vi "Finish.vi"   [LabVIEW 2017]
doc: "This VI is called just before exiting. It is expected to close I/O refnum, save collected data, etc."
uses:
  <vilib>/Rock Robotics/WPI/Utilities/WPI_GetSetVariantRefNum.vi
types:
  T1 = typedef "WPI_JoystickDevRef.ctl" = cluster{"Device":T2}
  T2 = typedef "WPI_JoystickDeviceEnum.ctl" = enum16{"USB 0", "USB 1", "USB 2", "USB 3", "USB 4", "USB 5"}
  T3 = typedef "WPI_DigitalInputDevRef.ctl" = cluster{"DevStatus":errorcluster, "DIO Channel":T4}
  T4 = typedef "FPGA_DIOChannel.ctl" = enum8{"DIO 0", "DIO 1", "DIO 2", "DIO 3", "DIO 4", "DIO 5", "DIO 6", "DIO 7", "DIO 8", "DIO 9", "DIO MXP 0", "DIO MXP 1", "DIO MXP 2", "DIO MXP 3", "DIO MXP 4", "DIO MXP 5", "DIO MXP 6", "DIO MXP 7", "DIO MXP 8", "DIO MXP 9", "DIO MXP 10", "DIO MXP 11", "DIO MXP 12", "DIO MXP 13", "DIO MXP 14", "DIO MXP 15", "SPI Port CS1", "SPI Port CS2", "SPI Port CS3", "SPI Port MISO", "SPI Port MOSI", "Invalid"}
  T5 = typedef "WPI_RobotDriveDevRef.ctl" = cluster{"DevStatus":errorcluster, "Motors[]":T6[], "Square Inputs":bool, "Max Output":dbl}
  T6 = typedef "WPI_MotorControlDeviceRef.ctl" = cluster{"DeviceStatus":errorcluster, "Type":T7, "PWM":cluster{"PWM Channel":T8, "DeadBand":T9}, "CAN":cluster{"Device Number":u8, "SetOutput VI Ref":variant, "GetOutput VI Ref":variant, "Enable VI Ref":variant, "Disable VI Ref":variant, "Data":variant}, "Invert":bool, "DIO PWM":cluster{"PWM \"Enable\" Channel":T8, "DIOChannel":T4, "PWM Rate":dbl}}
  T7 = typedef "WPI_MotorControlType.ctl" = enum16{"PWM", "CAN", "DIO PWM"}
  T8 = typedef "FPGA_DIOPWMChannel.ctl" = enum8{"PWM 0", "PWM 1", "PWM 2", "PWM 3", "PWM 4", "PWM 5", "PWM 6", "PWM 7", "PWM 8", "PWM 9", "PWM MXP 0", "PWM MXP 1", "PWM MXP 2", "PWM MXP 3", "PWM MXP 4", "PWM MXP 5", "PWM MXP 6", "PWM MXP 7", "PWM MXP 8", "PWM MXP 9", "Invalid"}
  T9 = typedef "WPI_PWMDeadband.ctl" = cluster{"Name":string, "maxPositivePwm":i32, "minPositivePwm":i32, "centerPwm":i32, "maxNegativePwm":i32, "minNegativePwm":i32, "angularRange":u16}
  T10 = typedef "WPI_SolenoidDevRef.ctl" = cluster{"DevStatus":errorcluster, "Pneumatics Control Module":u8, "Forward Solenoid Channel":T11, "Reverse Solenoid Channel":T11}
  T11 = typedef "WPI_SolenoidChannel.ctl" = enum8{"Solenoid 0", "Solenoid 1", "Solenoid 2", "Solenoid 3", "Solenoid 4", "Solenoid 5", "Solenoid 6", "Solenoid 7", "Invalid"}
  T12 = typedef "WPI_EncoderDevRef.ctl" = cluster{"DevStatus":errorcluster, "EncoderIndex":T13, "CounterIndex":T14, "DistancePerCount":dbl, "Decoding Type":T15}
  T13 = typedef "FPGA_EncoderIdx.ctl" = enum8{"Enc 0", "Enc 1", "Enc 2", "Enc 3", "Enc 4", "Enc 5", "Enc 6", "Enc 7", "Invalid"}
  T14 = typedef "FPGA_CounterCtrSystemIndex.ctl" = enum8{"Ctr 0", "Ctr 1", "Ctr 2", "Ctr 3", "Ctr 4", "Ctr 5", "Ctr 6", "Ctr 7", "Invalid"}
  T15 = typedef "WPI_EncoderType.ctl" = enum16{"1x", "2x", "4x"}
  T16 = typedef "WPI_CompressorDevRef.ctl" = cluster{"DevStatus":errorcluster, "Pneumatics Control Module":u8}
  T17 = typedef "WPI_SwitchDevRef.ctl" = cluster{"DevStatus":errorcluster, "DIO Channel":T4, "CntIndex":T14, "Normally Closed":bool}
  T18 = typedef "WPI_GyroDevRef.ctl" = cluster{"DevStatus":errorcluster, "Analog Channel":T19, "Gain (VoltsPerDegree/Second)":dbl, "Gyro Type":enum16{"Analog", "XRS450"}, "Handle":i32, "SPI Bus":T20, "Device Found":bool, "Sample Rate":dbl, "Calibrate On Open":bool, "Offset":dbl}
  T19 = typedef "FPGA_AIChannel.ctl" = enum8{"AI 0", "AI 1", "AI 2", "AI 3", "AI MXP 0", "AI MXP 1", "AI MXP 2", "AI MXP 3", "Invalid"}
  T20 = typedef "spi_bus.ctl" = enum16{"SPI On-Board, CS0", "SPI On-Board, CS1", "SPI On-Board, CS2", "SPI On-Board, CS3", "SPI MXP", "Invalid"}
  T21 = typedef "WPI_RelayDevRef.ctl" = cluster{"DevStatus":errorcluster, "Relay Channel":T22, "Relay Direction":T23}
  T22 = typedef "FPGA_DIORelayChannel.ctl" = enum8{"Relay 0", "Relay 1", "Relay 2", "Relay 3", "Invalid"}
  T23 = typedef "WPI_RelayDirection.ctl" = enum16{"Both directions", "Forward only", "Reverse only"}
  T24 = typedef "WPI_AnalogChannelDevRef.ctl" = cluster{"DevStatus":errorcluster, "Analog Channel":T19}
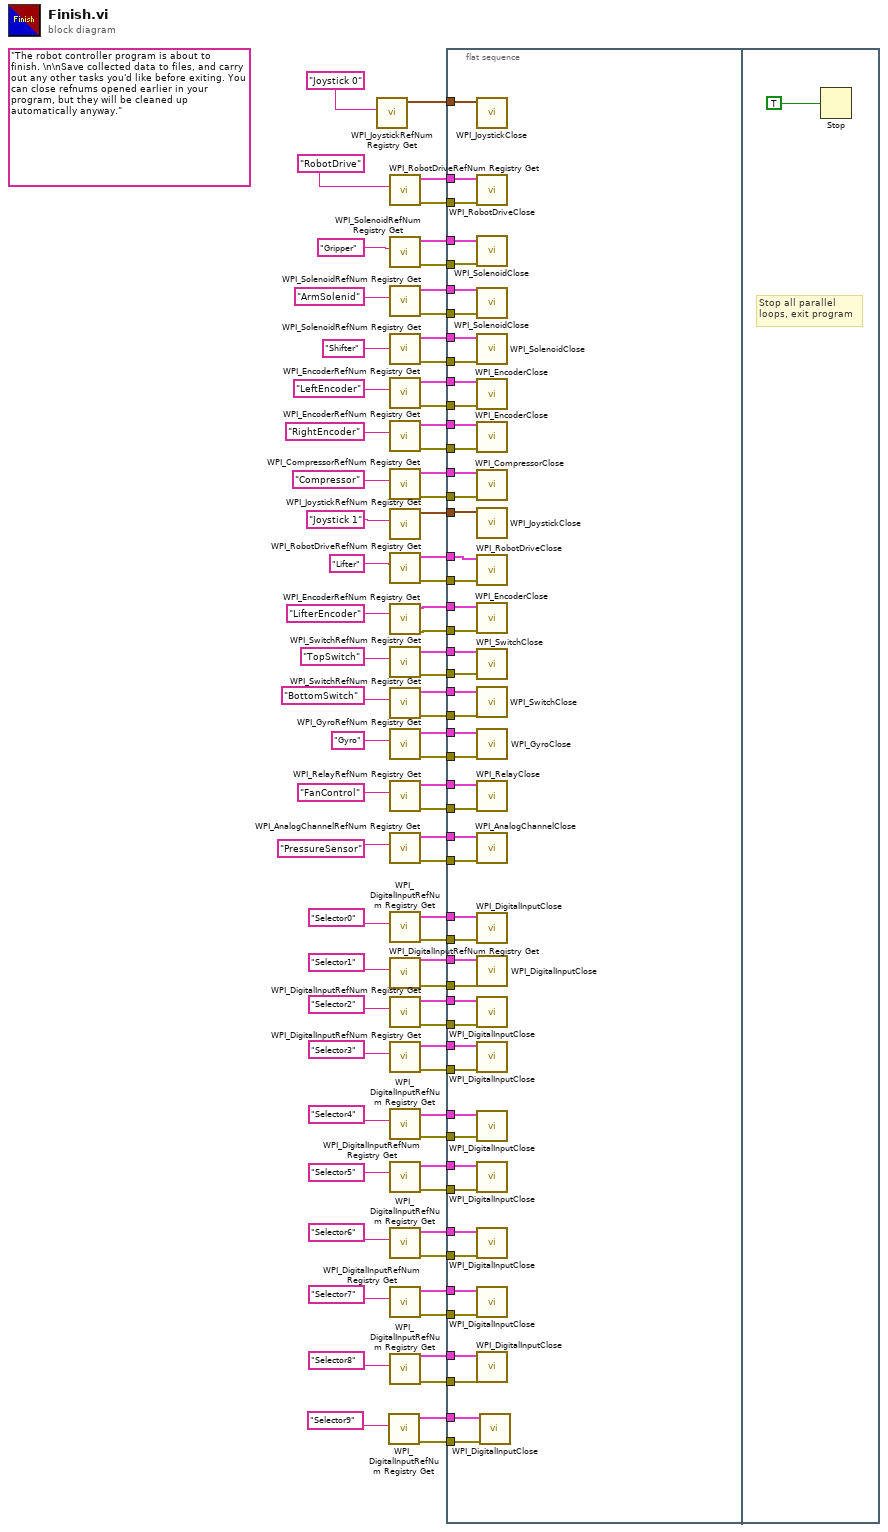
[diagram p0: block diagram]
diagram:
  (unwired) "The robot controller program is about to finish. \n\nSave collected data to files, and carry out any other tasks you'd like before exiting. You can close refnums opened earlier in your program, but they will be cleaned up automatically anyway."
  n1 = call <vilib>:"WPI_JoystickRefNum Registry Get.vi"("refnum name"="Joystick 0") -> ("JoystickDevRef"=w73:T1)  [unwired: 1 in, 9 out]
  n2 = call <vilib>:"WPI_DigitalInputRefNum Registry Get.vi"("refnum name"="Selector9") -> ("error out"=w1:errorcluster, "DigitalInputDevRef"=w2:T3)  [unwired: 9 in]
  n3 = call <vilib>:"WPI_RobotDriveRefNum Registry Get.vi"("refnum name"="RobotDrive") -> ("error out"=w34:errorcluster, "RobotDriveDevRef"=w74:T5)  [unwired: 1 in, 8 out]
  n4 = call <vilib>:"WPI_SolenoidRefNum Registry Get.vi"("refnum name"="Gripper") -> ("error out"=w65:errorcluster, "SolenoidDevRef"=w64:T10)  [unwired: 9 in]
  n5 = call <vilib>:"WPI_SolenoidRefNum Registry Get.vi"("refnum name"="ArmSolenid") -> ("error out"=w67:errorcluster, "SolenoidDevRef"=w66:T10)  [unwired: 9 in]
  n6 = call <vilib>:"WPI_SolenoidRefNum Registry Get.vi"("refnum name"="Shifter") -> ("error out"=w69:errorcluster, "SolenoidDevRef"=w68:T10)  [unwired: 9 in]
  n7 = call <vilib>:"WPI_EncoderRefNum Registry Get.vi"("refnum name"="LeftEncoder") -> ("error out"=w63:errorcluster, "EncoderDevRef"=w62:T12)  [unwired: 9 in]
  n8 = call <vilib>:"WPI_EncoderRefNum Registry Get.vi"("refnum name"="RightEncoder") -> ("error out"=w61:errorcluster, "EncoderDevRef"=w60:T12)  [unwired: 9 in]
  n9 = call <vilib>:"WPI_CompressorRefNum Registry Get.vi"("refnum name"="Compressor") -> ("error out"=w57:errorcluster, "CompressorDevRef"=w56:T16)  [unwired: 9 in]
  n10 = call <vilib>:"WPI_JoystickRefNum Registry Get.vi"("refnum name"="Joystick 1") -> ("JoystickDevRef"=w53:T1)  [unwired: 9 in, 1 out]
  n11 = call <vilib>:"WPI_RobotDriveRefNum Registry Get.vi"("refnum name"="Lifter") -> ("error out"=w35:errorcluster, "RobotDriveDevRef"=w52:T5)  [unwired: 9 in]
  n12 = call <vilib>:"WPI_EncoderRefNum Registry Get.vi"("refnum name"="LifterEncoder") -> ("error out"=w48:errorcluster, "EncoderDevRef"=w49:T12)  [unwired: 9 in]
  n13 = call <vilib>:"WPI_SwitchRefNum Registry Get.vi"("refnum name"="TopSwitch") -> ("error out"=w46:errorcluster, "SwitchDevRef"=w47:T17)  [unwired: 9 in]
  n14 = call <vilib>:"WPI_SwitchRefNum Registry Get.vi"("refnum name"="BottomSwitch") -> ("error out"=w43:errorcluster, "SwitchDevRef"=w44:T17)  [unwired: 9 in]
  n15 = call <vilib>:"WPI_GyroRefNum Registry Get.vi"("refnum name"="Gyro") -> ("error out"=w41:errorcluster, "GyroDevRef"=w40:T18)  [unwired: 9 in]
  n16 = call <vilib>:"WPI_RelayRefNum Registry Get.vi"("refnum name"="FanControl") -> ("error out"=w37:errorcluster, "RelayDevRef"=w38:T21)  [unwired: 9 in]
  n17 = call <vilib>:"WPI_AnalogChannelRefNum Registry Get.vi"("refnum name"="PressureSensor") -> ("error out"=w31:errorcluster, "AIDeviceRef"=w32:T24)  [unwired: 9 in]
  n18 = call <vilib>:"WPI_DigitalInputRefNum Registry Get.vi"("refnum name"="Selector0") -> ("error out"=w29:errorcluster, "DigitalInputDevRef"=w30:T3)  [unwired: 9 in]
  n19 = call <vilib>:"WPI_DigitalInputRefNum Registry Get.vi"("refnum name"="Selector1") -> ("error out"=w18:errorcluster, "DigitalInputDevRef"=w19:T3)  [unwired: 9 in]
  n20 = call <vilib>:"WPI_DigitalInputRefNum Registry Get.vi"("refnum name"="Selector2") -> ("error out"=w16:errorcluster, "DigitalInputDevRef"=w17:T3)  [unwired: 9 in]
  n21 = call <vilib>:"WPI_DigitalInputRefNum Registry Get.vi"("refnum name"="Selector3") -> ("error out"=w14:errorcluster, "DigitalInputDevRef"=w15:T3)  [unwired: 9 in]
  n22 = call <vilib>:"WPI_DigitalInputRefNum Registry Get.vi"("refnum name"="Selector4") -> ("error out"=w12:errorcluster, "DigitalInputDevRef"=w13:T3)  [unwired: 9 in]
  n23 = call <vilib>:"WPI_DigitalInputRefNum Registry Get.vi"("refnum name"="Selector5") -> ("error out"=w10:errorcluster, "DigitalInputDevRef"=w11:T3)  [unwired: 9 in]
  n24 = call <vilib>:"WPI_DigitalInputRefNum Registry Get.vi"("refnum name"="Selector6") -> ("error out"=w8:errorcluster, "DigitalInputDevRef"=w9:T3)  [unwired: 9 in]
  n25 = call <vilib>:"WPI_DigitalInputRefNum Registry Get.vi"("refnum name"="Selector7") -> ("error out"=w6:errorcluster, "DigitalInputDevRef"=w7:T3)  [unwired: 9 in]
  n26 = call <vilib>:"WPI_DigitalInputRefNum Registry Get.vi"("refnum name"="Selector8") -> ("error out"=w4:errorcluster, "DigitalInputDevRef"=w5:T3)  [unwired: 9 in]
  n27 = flat-sequence {
    tunnel: w74 -> [w126]
    tunnel: w73 -> [w125]
    tunnel: w69 -> [w124]
    tunnel: w68 -> [w123]
    tunnel: w67 -> [w122]
    tunnel: w66 -> [w121]
    tunnel: w65 -> [w120]
    tunnel: w64 -> [w119]
    tunnel: w63 -> [w118]
    tunnel: w62 -> [w117]
    tunnel: w61 -> [w116]
    tunnel: w60 -> [w115]
    tunnel: w57 -> [w114]
    tunnel: w56 -> [w113]
    tunnel: w53 -> [w112]
    tunnel: w52 -> [w111]
    tunnel: w49 -> [w110]
    tunnel: w48 -> [w109]
    tunnel: w47 -> [w108]
    tunnel: w46 -> [w107]
    tunnel: w44 -> [w106]
    tunnel: w43 -> [w105]
    tunnel: w41 -> [w104]
    tunnel: w40 -> [w103]
    tunnel: w38 -> [w102]
    tunnel: w37 -> [w101]
    tunnel: w35 -> [w100]
    tunnel: w34 -> [w99]
    tunnel: w32 -> [w98]
    tunnel: w31 -> [w97]
    tunnel: w30 -> [w96]
    tunnel: w29 -> [w95]
    tunnel: w19 -> [w94]
    tunnel: w18 -> [w93]
    tunnel: w17 -> [w92]
    tunnel: w16 -> [w91]
    tunnel: w15 -> [w90]
    tunnel: w14 -> [w89]
    tunnel: w13 -> [w88]
    tunnel: w12 -> [w87]
    tunnel: w11 -> [w86]
    tunnel: w10 -> [w85]
    tunnel: w9 -> [w84]
    tunnel: w8 -> [w83]
    tunnel: w7 -> [w82]
    tunnel: w6 -> [w81]
    tunnel: w5 -> [w80]
    tunnel: w4 -> [w79]
    tunnel: w2 -> [w78]
    tunnel: w1 -> [w77]
    frame #0 {
      n28 = call <vilib>:"WPI_JoystickClose.vi"("JoystickDevRef"=w125) -> ()  [unwired: 11 out]
      n29 = call <vilib>:"WPI_RobotDriveClose.vi"("error in (no error)"=w99, "RobotDriveDevRef"=w126) -> ()  [unwired: 10 out]
      n30 = call <vilib>:"WPI_SolenoidClose.vi"("error in (no error)"=w120, "SolenoidDevRef"=w119) -> ()  [unwired: 9 in, 1 out]
      n31 = call <vilib>:"WPI_SolenoidClose.vi"("error in (no error)"=w122, "SolenoidDevRef"=w121) -> ()  [unwired: 9 in, 1 out]
      n32 = call <vilib>:"WPI_SolenoidClose.vi"("error in (no error)"=w124, "SolenoidDevRef"=w123) -> ()  [unwired: 9 in, 1 out]
      n33 = call <vilib>:"WPI_EncoderClose.vi"("error in (no error)"=w118, "EncoderDevRef"=w117) -> ()  [unwired: 9 in, 1 out]
      n34 = call <vilib>:"WPI_EncoderClose.vi"("error in (no error)"=w116, "EncoderDevRef"=w115) -> ()  [unwired: 9 in, 1 out]
      n35 = call <vilib>:"WPI_CompressorClose.vi"("error in (no error)"=w114, "CompressorDevRef"=w113) -> ()  [unwired: 9 in, 1 out]
      n36 = call <vilib>:"WPI_JoystickClose.vi"("JoystickDevRef"=w112) -> ()  [unwired: 11 out]
      n37 = call <vilib>:"WPI_RobotDriveClose.vi"("error in (no error)"=w100, "RobotDriveDevRef"=w111) -> ()  [unwired: 9 in, 1 out]
      n38 = call <vilib>:"WPI_EncoderClose.vi"("error in (no error)"=w109, "EncoderDevRef"=w110) -> ()  [unwired: 9 in, 1 out]
      n39 = call <vilib>:"WPI_SwitchClose.vi"("error in (no error)"=w107, "SwitchDevRef"=w108) -> ()  [unwired: 9 in, 1 out]
      n40 = call <vilib>:"WPI_SwitchClose.vi"("error in (no error)"=w105, "SwitchDevRef"=w106) -> ()  [unwired: 9 in, 1 out]
      n41 = call <vilib>:"WPI_GyroClose.vi"("error in"=w104, "GyroDevRef"=w103) -> ()  [unwired: 9 in, 1 out]
      n42 = call <vilib>:"WPI_RelayClose.vi"("error in (no error)"=w101, "RelayDevRef"=w102) -> ()  [unwired: 9 in, 1 out]
      n43 = call <vilib>:"WPI_AnalogChannelClose.vi"("error in (no error)"=w97, "AIDeviceRef"=w98) -> ()  [unwired: 9 in, 1 out]
      n44 = call <vilib>:"WPI_DigitalInputClose.vi"("error in (no error)"=w95, "DigitalInputDevRef"=w96) -> ()  [unwired: 9 in, 1 out]
      n45 = call <vilib>:"WPI_DigitalInputClose.vi"("error in (no error)"=w93, "DigitalInputDevRef"=w94) -> ()  [unwired: 9 in, 1 out]
      n46 = call <vilib>:"WPI_DigitalInputClose.vi"("error in (no error)"=w91, "DigitalInputDevRef"=w92) -> ()  [unwired: 9 in, 1 out]
      n47 = call <vilib>:"WPI_DigitalInputClose.vi"("error in (no error)"=w89, "DigitalInputDevRef"=w90) -> ()  [unwired: 9 in, 1 out]
      n48 = call <vilib>:"WPI_DigitalInputClose.vi"("error in (no error)"=w87, "DigitalInputDevRef"=w88) -> ()  [unwired: 9 in, 1 out]
      n49 = call <vilib>:"WPI_DigitalInputClose.vi"("error in (no error)"=w85, "DigitalInputDevRef"=w86) -> ()  [unwired: 9 in, 1 out]
      n50 = call <vilib>:"WPI_DigitalInputClose.vi"("error in (no error)"=w83, "DigitalInputDevRef"=w84) -> ()  [unwired: 9 in, 1 out]
      n51 = call <vilib>:"WPI_DigitalInputClose.vi"("error in (no error)"=w81, "DigitalInputDevRef"=w82) -> ()  [unwired: 9 in, 1 out]
      n52 = call <vilib>:"WPI_DigitalInputClose.vi"("error in (no error)"=w79, "DigitalInputDevRef"=w80) -> ()  [unwired: 9 in, 1 out]
      n53 = call <vilib>:"WPI_DigitalInputClose.vi"("error in (no error)"=w77, "DigitalInputDevRef"=w78) -> ()  [unwired: 9 in, 1 out]
    }
    frame #1 {
      # "Stop all parallel\nloops, exit program"
      n54 = Stop(stop? (T)=TRUE ("Quit")) -> ()
    }
  }
